vi "Config to DB Data.vi"(8 "error in (no error)":errorcluster, 11 "Control References Array":refnum<vi>[](array[refnum])) -> (0 "error out":errorcluster, 2 "Name":string[](array[string]), 3 "Data":string[](array[string]))   [LabVIEW 2017]
panel:
  out "Array":u32[](array[numeric])
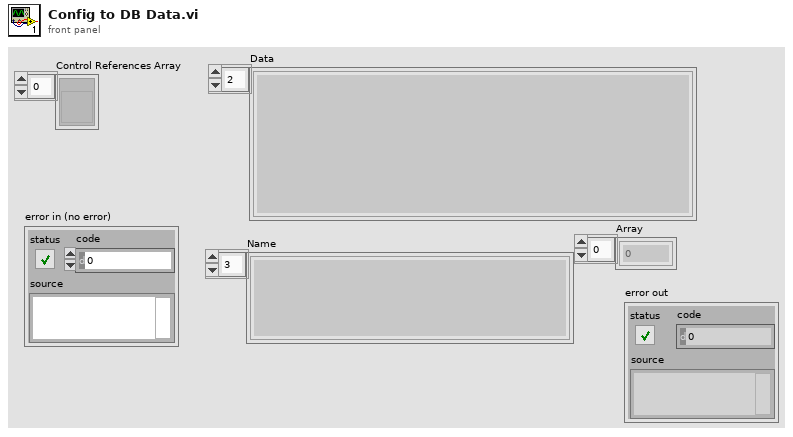
[diagram p1: front panel]
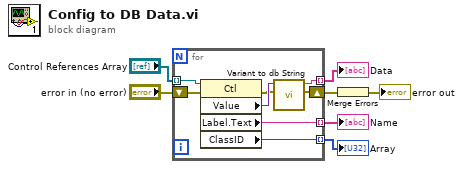
[diagram p0: block diagram]
diagram:
  n1 = for {
    tunnel: "Control References Array" -> [w15] mode=indexing
    tunnel: [w12] -> w6 mode=indexing
    tunnel: [w14] -> w5 mode=indexing
    tunnel: [w13] -> w4 mode=indexing
    shift-right: [w8] -> w2
    shift-left: "error in (no error)" -> [w9]
    n2 = property class="Ctl"(reference=w15, error in=w9) -> (error out=w10:errorcluster, "Value"=w11:variant, "Label.Text"=w14:string, "ClassID"=w13:u32)  [unwired: 1 out]
    n3 = call "Variant to db String.vi"("error in (no error)"=w10, "Control Data"=w11) -> ("error out"=w8:errorcluster, "DB String"=w12:string)  [unwired: 7 in, 1 out]
  }
  "Data" <- w6
  "Name" <- w5
  "Array" <- w4
  n4 = Merge Errors(w2) -> (→"error out":errorcluster)
